vi "Configure Config Session.vi"(8 "error in":errorcluster, 9 "Path":path, 10 "Ref Name":string, 11 "Configurable Device in":refnum<class "Configurable Device.lvclass">) -> (0 "error out":errorcluster, 3 "Configurable Device out":refnum<class "Configurable Device.lvclass">)   [LabVIEW 2014, in "Device.lvlib" / "Configurable Device.lvclass"]
uses:
  Configurable Device.lvclass
  reusable/Session APIs/File Access/Config Data/Config Data.lvclass
  reusable/Session APIs/File Access/Config Data/Config Data.lvclass/Config Data.ctl
  Configurable Device.lvclass/Configurable Device.ctl
  reusable/Session APIs/File Access/Config Data/Accessors/Write Cfg Path.vi
  <userlib>/_Session Fwk/Session - Root.lvclass
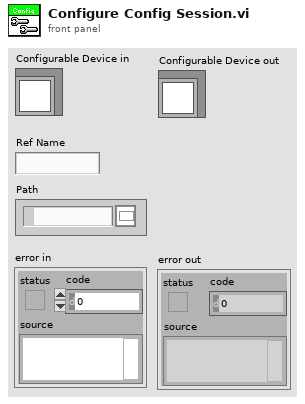
[diagram p1: front panel]
types:
  T1 = typedef "Session - Root.lvclass/Session Handle.ctl" = refnum<data-value>
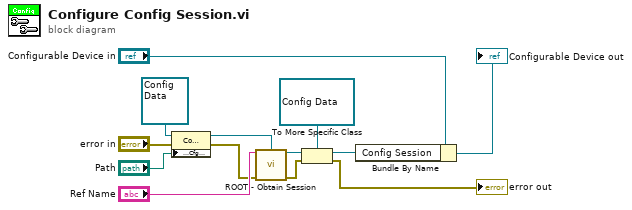
[diagram p0: block diagram]
diagram:
  n1 = property class="Config Data"(reference=refnum<class "Config Data.lvclass"> refnum ("Config Data"), error in="error in", "Accessors:Cfg Path"="Path") -> (reference out=w11:refnum<class "Config Data.lvclass">, error out=w9:errorcluster)
  n2 = call <userlib>:"ROOT - Obtain Session.vi"("Session Name ()"="Ref Name", "OBJ - Session"=w11, "error in (no error)"=w9) -> ("Session Handle"=w5:T1, "error out"=w2:errorcluster)  [unwired: 10 in, 1 out]
  n3 = To More Specific Class(target class=refnum<data-value> refnum, reference=w5, error in=w2) -> (specific class reference=w4:refnum<data-value>, error out=→"error out":errorcluster)
  n4 = Bundle By Name(cluster="Configurable Device in", "Config Session"=w4) -> (→"Configurable Device out":refnum<class "Configurable Device.lvclass">)
